vi "Wind Turbine Object Snooper.vi"() -> ()   [LabVIEW 2009, in "SEQ - Solution.lvlib"]
doc: "One VI in the solution for the Wind Turbine class. This group of VIs is built on the SEQ design pattern and illustrates the power of references and named queues.\n\nAAL 9/09"
uses:
  SEQ - Solution.lvlib
  Controls/Wind Turbine Data.ctl
panel:
  out "Data":T1
  in  "SEQ Name":string
  in  "Update Time (ms)":u32=100
  in  "stop":bool
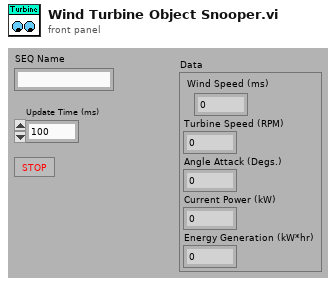
[diagram p1: front panel]
types:
  T1 = typedef "SEQ - Solution.lvlib/Wind Turbine Data.ctl" = cluster{" Wind Speed (ms)":dbl, "Turbine Speed (RPM)":dbl, "Angle Attack (Degs.)":dbl, "Current Power (kW)":dbl, "Energy Generation (kW*hr)":dbl}
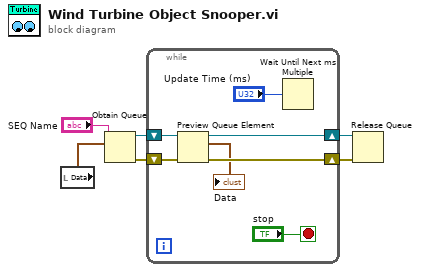
[diagram p0: block diagram]
diagram:
  n1 = local read "Data"() -> (w3:T1)
  n2 = Obtain Queue(name (unnamed)="SEQ Name", element data type=w3) -> (queue out=w4:refnum<queue>, error out=w5:errorcluster)  [unwired: 3 in, 1 out]
  n3 = while {
    shift-right: [w9] -> w2
    shift-left: w5 -> [w11]
    shift-right: [w7] -> w1
    shift-left: w4 -> [w10]
    stop <- "stop" stop-if-true
    n4 = Preview Queue Element(queue=w10, error in (no error)=w11) -> (queue out=w7:refnum<queue>, element=→"Data":T1, error out=w9:errorcluster)  [unwired: 2 out]
    n5 = Wait Until Next ms Multiple(millisecond multiple="Update Time (ms)") -> ()  [unwired: 1 out]
  }
  n6 = Release Queue(queue=w1, error in (no error)=w2) -> ()  [unwired: 4 out]
